vi "Format Variant.vi"(1 "Raw Variant":variant) -> (0 "Formatted Variant":variant)   [LabVIEW 2017, in "TreeLUT.lvclass"]
uses:
  TreeLUT.lvclass
  <vilib>/vision/Image Controls.llb/IMAQ Image.ctl
  <vilib>/Utility/Data Type/NI_Data Type.lvlib
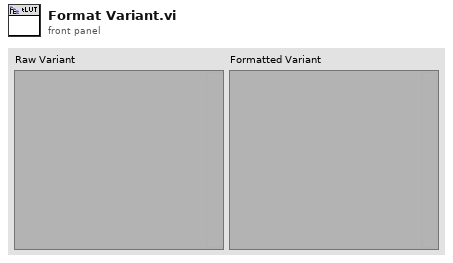
[diagram p1: front panel]
types:
  T1 = typedef "NI_Data Type.lvlib/Data Type.ctl" = enum8{"Invalid Type", "Void", "I8", "I16", "I32", "I64", "U8", "U16", "U32", "U64", "Single Float", "Double Float", "Extended Float", "Single Complex", "Double Complex", "Extended Complex", "Enum U8", "Enum U16", "Enum U32", "Enum U64", "Single Float With Unit", "Double Float With Unit", "Extended Float With Unit", "Single Complex with Unit", "Double Complex with Unit", "Extended Complex with Unit", "Boolean", "String", "Path", "Picture", "Tag", "Array", "Cluster", "Variant", "LV Variant", "Waveform", "Timestamp", "Digital Waveform", "Digital Data", "ExpressData", "Refnum", "External Data", "VI", "Poly VI", "LabVIEW Class Instance", "Fixed Point"}
  T2 = typedef "IMAQ Image.ctl" = refnum<image>
  T3 = typedef "NI_Data Type.lvlib/Type Definition Info.ctl" = cluster{"Name":string, "Timestamp":u32}
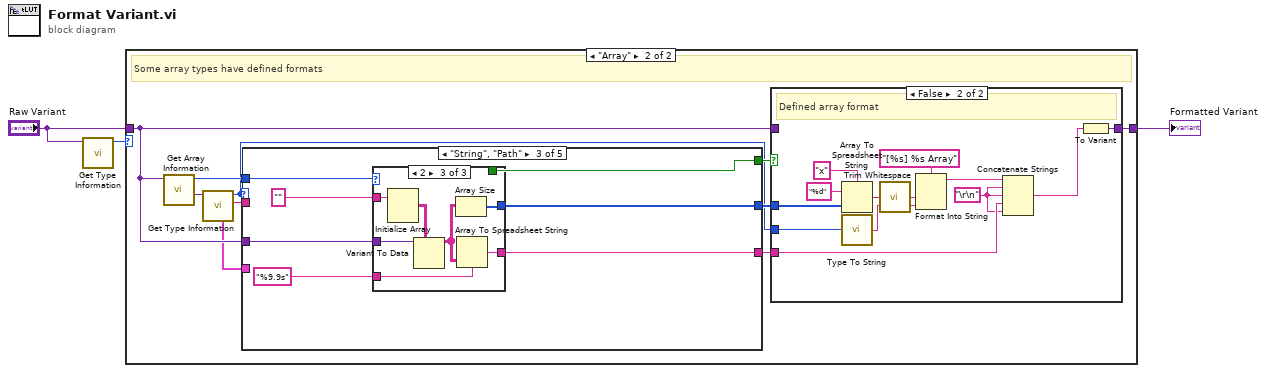
[diagram p0: block diagram]
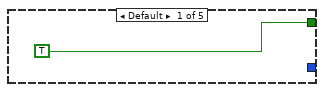
[diagram p4: hidden frame]
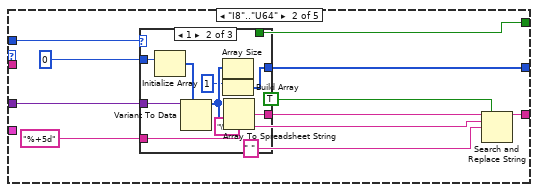
[diagram p5: hidden frame]
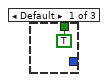
[diagram p6: hidden frame]
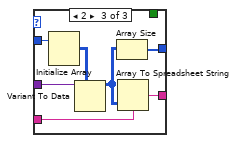
[diagram p7: hidden frame]
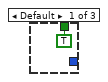
[diagram p8: hidden frame]
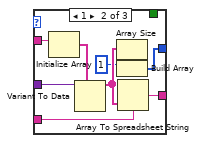
[diagram p9: hidden frame]
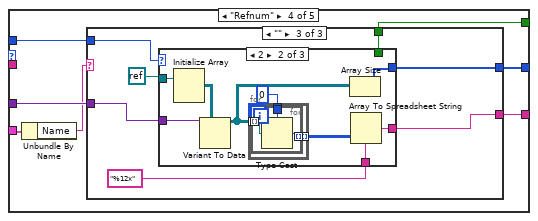
[diagram p10: hidden frame]
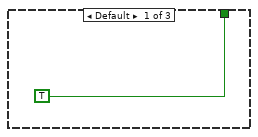
[diagram p11: hidden frame]
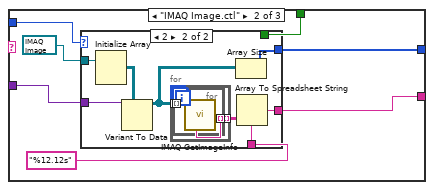
[diagram p12: hidden frame]
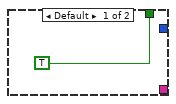
[diagram p13: hidden frame]
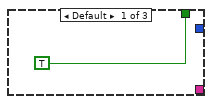
[diagram p14: hidden frame]
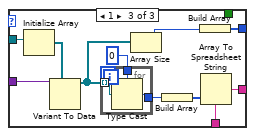
[diagram p15: hidden frame]
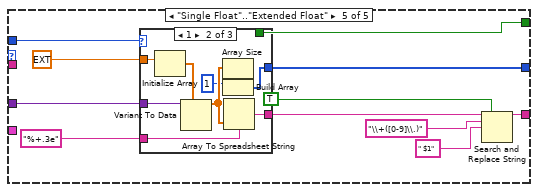
[diagram p16: hidden frame]
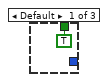
[diagram p17: hidden frame]
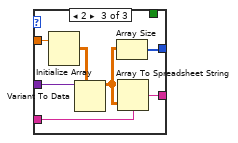
[diagram p18: hidden frame]
diagram:
  n1 = call <vilib>:"Get Type Information.vi"("Variant"="Raw Variant") -> ("Type"=w1:T1)  [unwired: 6 in, 4 out]
  n2 = case shown="\"Array\"" w1 {
    tunnel: "Raw Variant" -> [w4 w9]
    tunnel: [w4 w11] -> w3
    frame Default {
      # "Undefined format"
    }
    frame "Array" {
      # "Some array types have defined formats"
      n3 = call <vilib>:"Get Array Information.vi"("Variant"=w9) -> ("Array Element Data Type"=w14:variant, "Number of Dimensions"=w13:i32)  [unwired: 7 in, 2 out]
      n4 = call <vilib>:"Get Type Information.vi"("Variant"=w14) -> ("Name"=w7:string, "Type"=w5:T1, "Type Definition Info"=w6:T3)  [unwired: 6 in, 2 out]
      n5 = case shown="\"String\", \"Path\"" w5 {
        tunnel: w13 -> [_ w39 w63 w88 w156]
        tunnel: w9 -> [_ w38 w62 w87 w155]
        tunnel: [_ w36 w60 w85 w153] -> w12
        tunnel: [_ w33 w58 w84 w150] -> w8
        tunnel: [TRUE w35 w59 w86 w152] -> w10
        tunnel: w7 -> [_ _ _ _ _]
        tunnel: w6 -> [_ _ _ w83 _]
        frame Default {
        }
        frame "I8".."U64" {
          n6 = case shown="1" w39 {
            tunnel: i64 0 -> [_ w50 w57]
            tunnel: w38 -> [_ w48 w55]
            tunnel: [_ w46 w51] -> w36
            tunnel: [_ w44 w53] -> w34
            tunnel: "%+5d" -> [_ w43 w52]
            tunnel: [TRUE _ _] -> w35
            frame Default {
            }
            frame 1 {
              n7 = Initialize Array(w50) -> (w49:i64[])  [unwired: 1 in]
              n8 = Variant To Data(type=w49, Variant=w48) -> (data=w45:i64[])  [unwired: 1 in, 1 out]
              n9 = Array Size(array=w45) -> (size(s)=w47:i32)
              n10 = Build Array(1 ("element"), w47) -> (w46:i32[])
              n11 = Array To Spreadsheet String(array=w45, 3:w43) -> (spreadsheet string=w44:string)  [unwired: 1 in]
            }
            frame 2 {
              n12 = Initialize Array(w57) -> (w56:i64[][])  [unwired: 2 in]
              n13 = Variant To Data(type=w56, Variant=w55) -> (data=w54:i64[][])  [unwired: 1 in, 1 out]
              n14 = Array Size(array=w54) -> (size(s)=w51:i32[])
              n15 = Array To Spreadsheet String(array=w54, 3:w52) -> (spreadsheet string=w53:string)  [unwired: 1 in]
            }
          }
          n16 = Search and Replace String(replace all?=TRUE ("replace all? (F)"), input string=w34, search string="\\+", replace string=" ") -> (result string=w33:string)  [unwired: 4 in, 3 out]
        }
        frame "String", "Path" {
          n17 = case shown="2" w63 {
            tunnel: "" -> [_ w74 w81]
            tunnel: w62 -> [_ w72 w79]
            tunnel: [_ w70 w75] -> w60
            tunnel: [_ w68 w77] -> w58
            tunnel: "%9.9s" -> [_ w67 w76]
            tunnel: [TRUE _ _] -> w59
            frame Default {
            }
            frame 1 {
              n18 = Initialize Array(w74) -> (w73:string[])  [unwired: 1 in]
              n19 = Variant To Data(type=w73, Variant=w72) -> (data=w69:string[])  [unwired: 1 in, 1 out]
              n20 = Array Size(array=w69) -> (size(s)=w71:i32)
              n21 = Build Array(1 ("element"), w71) -> (w70:i32[])
              n22 = Array To Spreadsheet String(array=w69, 3:w67) -> (spreadsheet string=w68:string)  [unwired: 1 in]
            }
            frame 2 {
              n23 = Initialize Array(w81) -> (w80:string[][])  [unwired: 2 in]
              n24 = Variant To Data(type=w80, Variant=w79) -> (data=w78:string[][])  [unwired: 1 in, 1 out]
              n25 = Array Size(array=w78) -> (size(s)=w75:i32[])
              n26 = Array To Spreadsheet String(array=w78, 3:w76) -> (spreadsheet string=w77:string)  [unwired: 1 in]
            }
          }
        }
        frame "Refnum" {
          n27 = Unbundle By Name(w83) -> ("Name"=w82:string)
          n28 = case shown="\"\"" w82 {
            tunnel: w88 -> [_ w96 w116]
            tunnel: w87 -> [_ w95 w115]
            tunnel: [TRUE w92 w114] -> w86
            tunnel: [_ w91 w113] -> w85
            tunnel: [_ w90 w112] -> w84
            frame Default {
            }
            frame "IMAQ Image.ctl" {
              n29 = case shown="2" w96 {
                tunnel: [_ w105] -> w90
                tunnel: [TRUE _] -> w92
                tunnel: T2 refnum ("Image") -> [_ w104]
                tunnel: w95 -> [_ w103]
                tunnel: "%12.12s" -> [_ w102]
                tunnel: [_ w98] -> w91
                frame Default {
                }
                frame 2 {
                  n30 = Initialize Array(w104) -> (w101:T2[][])  [unwired: 2 in]
                  n31 = Variant To Data(type=w101, Variant=w103) -> (data=w100:T2[][])  [unwired: 1 in, 1 out]
                  n32 = for {
                    tunnel: w100 -> [w107] mode=indexing
                    tunnel: [w106] -> w99 mode=indexing
                    n33 = for {
                      tunnel: w107 -> [w109] mode=indexing
                      tunnel: [w108] -> w106 mode=indexing
                      n34 = call "IMAQ GetImageInfo"("Image"=w109) -> ("Image Name"=w108:string)  [unwired: 3 in, 7 out]
                    }
                  }
                  n35 = Array Size(array=w100) -> (size(s)=w98:i32[])
                  n36 = Array To Spreadsheet String(array=w99, 3:w102) -> (spreadsheet string=w105:string)  [unwired: 1 in]
                }
              }
            }
            frame "" {
              n37 = case shown="2" w116 {
                tunnel: [_ w126 w143] -> w112
                tunnel: [TRUE _ _] -> w114
                tunnel: refnum<k0> refnum -> [_ w125 w142]
                tunnel: w115 -> [_ w124 w141]
                tunnel: "%12x" -> [_ w123 w140]
                tunnel: [_ w119 w134] -> w113
                frame Default {
                }
                frame 2 {
                  n38 = Initialize Array(w125) -> (w122:refnum<k0>[][])  [unwired: 2 in]
                  n39 = Variant To Data(type=w122, Variant=w124) -> (data=w121:refnum<k0>[][])  [unwired: 1 in, 1 out]
                  n40 = for {
                    tunnel: w121 -> [w128] mode=indexing
                    tunnel: [w129] -> w120 mode=indexing
                    tunnel: 0 -> [w127]
                    n41 = for {
                      tunnel: [w132] -> w129 mode=indexing
                      tunnel: w128 -> [w131] mode=indexing
                      tunnel: w127 -> [w130]
                      n42 = Type Cast(type=w130, x=w131) -> (*(type *) &x=w132:i32)
                    }
                  }
                  n43 = Array Size(array=w121) -> (size(s)=w119:i32[])
                  n44 = Array To Spreadsheet String(array=w120, 3:w123) -> (spreadsheet string=w126:string)  [unwired: 1 in]
                }
                frame 1 {
                  n45 = Initialize Array(w142) -> (w139:refnum<k0>[])  [unwired: 1 in]
                  n46 = Variant To Data(type=w139, Variant=w141) -> (data=w138:refnum<k0>[])  [unwired: 1 in, 1 out]
                  n47 = for {
                    tunnel: [w146] -> w137
                    tunnel: w138 -> [w145] mode=indexing
                    tunnel: i64 0 -> [w144]
                    n48 = Type Cast(type=w144, x=w145) -> (*(type *) &x=w146:i64)
                  }
                  n49 = Array Size(array=w138) -> (size(s)=w136:i32)
                  n50 = Build Array(w137) -> (w133:i64[])
                  n51 = Build Array(w136) -> (w134:i32[])
                  n52 = Array To Spreadsheet String(array=w133, 3:w140) -> (spreadsheet string=w143:string)  [unwired: 1 in]
                }
              }
            }
          }
        }
        frame "Single Float".."Extended Float" {
          n53 = case shown="1" w156 {
            tunnel: ext 0.0 -> [_ w167 w174]
            tunnel: w155 -> [_ w165 w172]
            tunnel: [_ w163 w168] -> w153
            tunnel: [_ w161 w170] -> w151
            tunnel: "%+.3e" -> [_ w160 w169]
            tunnel: [TRUE _ _] -> w152
            frame Default {
            }
            frame 1 {
              n54 = Initialize Array(w167) -> (w166:ext[])  [unwired: 1 in]
              n55 = Variant To Data(type=w166, Variant=w165) -> (data=w162:ext[])  [unwired: 1 in, 1 out]
              n56 = Array Size(array=w162) -> (size(s)=w164:i32)
              n57 = Build Array(1 ("element"), w164) -> (w163:i32[])
              n58 = Array To Spreadsheet String(array=w162, 3:w160) -> (spreadsheet string=w161:string)  [unwired: 1 in]
            }
            frame 2 {
              n59 = Initialize Array(w174) -> (w173:ext[][])  [unwired: 2 in]
              n60 = Variant To Data(type=w173, Variant=w172) -> (data=w171:ext[][])  [unwired: 1 in, 1 out]
              n61 = Array Size(array=w171) -> (size(s)=w168:i32[])
              n62 = Array To Spreadsheet String(array=w171, 3:w169) -> (spreadsheet string=w170:string)  [unwired: 1 in]
            }
          }
          n63 = Search and Replace String(replace all?=TRUE ("replace all? (F)"), input string=w151, search string="\\+([0-9]\\.)", replace string=" $1") -> (result string=w150:string)  [unwired: 4 in, 3 out]
        }
      }
      n64 = case shown="False" w10 {
        tunnel: w12 -> [_ w23]
        tunnel: [w15 w22] -> w11
        tunnel: w9 -> [w15 _]
        tunnel: w8 -> [_ w20]
        tunnel: w5 -> [_ w16]
        frame True {
          # "Undefined array format"
        }
        frame False {
          w18 = "\r\n"
          # "Defined array format"
          n65 = Array To Spreadsheet String(delimiter (Tab)="x", array=w23, 3:"%d") -> (spreadsheet string=w25:string)
          n66 = call "Type To String.vi"("Data Type"=w16) -> ("Data Type String"=w17:string)  [unwired: 14 in]
          n67 = call <vilib>:"Trim Whitespace.vi"("string"=w25) -> ("trimmed string"=w24:string)  [unwired: 1 in]
          n68 = Format Into String(format string="[%s] %s Array", w24, w17) -> (resulting string=w21:string)  [unwired: 2 in, 1 out]
          n69 = Concatenate Strings(w21, w18, w18, w20, w18) -> (w19:string)
          n70 = To Variant(anything=w19) -> (Variant=w22:variant)
        }
      }
    }
  }
  "Formatted Variant" <- w3
